vi "Error Query.vi"(6 "Ignored Warnings":string[](array[string]), 7 "Warnings as Errors":string[](array[string]), 8 "error in (no error)":errorcluster, 9 "Device and Axis":string, 10 "Previous Response Bundle Array":T1(array[cluster]), 11 "VISA resource name":refnum<visa-resource-name>) -> (0 "error out":errorcluster, 1 "Error Message":string, 2 "Error Code":i32, 3 "VISA resource name out":refnum<visa-resource-name>)   [LabVIEW 2015, in "Zaber A Series.lvlib"]
doc: "Checks a collection of responses for warning flags and reports all warnings from responding devices that have warning conditions.\n\nOptional inputs allow for ignoring some warnings or treating some warnings as error conditions. Both of these inputs are arrays of strings, each of which should be a two-letter warning code as seen in the Zaber ASCII Protocol Manual at http://www.zaber.com/wiki/Manuals/ASCII_Protocol_Manual#Warning_Flags. \n\nYou can globally ignore warnings or treat warnings as errors without having to wire up the relevant inputs everywhere by entering new defaults for the inputs - see the note on this VI's front panel.\n\nThis VI requires that the Initialize VI has been called with the same serial port."
uses:
  Zaber A Series.lvlib
  Private/All Commands.ctl
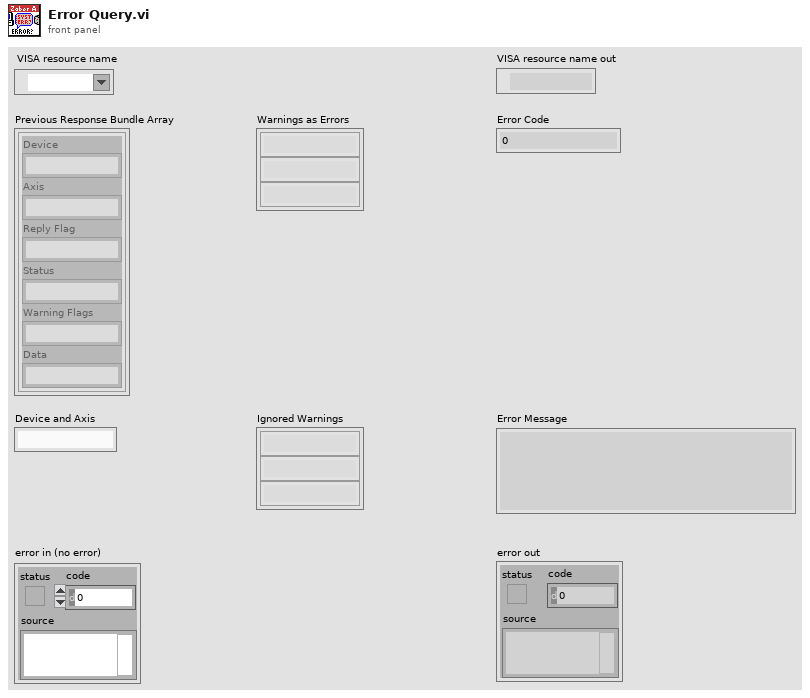
[diagram p1: front panel]
types:
  T1 = cluster{"Device":string, "Axis":string, "Reply Flag":string, "Status":string, "Warning Flags":string, "Data":string}[]
  T2 = typedef "Zaber A Series.lvlib/All Commands.ctl" = string
  T3 = cluster{"Device":string, "Axis":string, "Reply Flag":string, "Status":string, "Warning Flags":string, "Data":string}
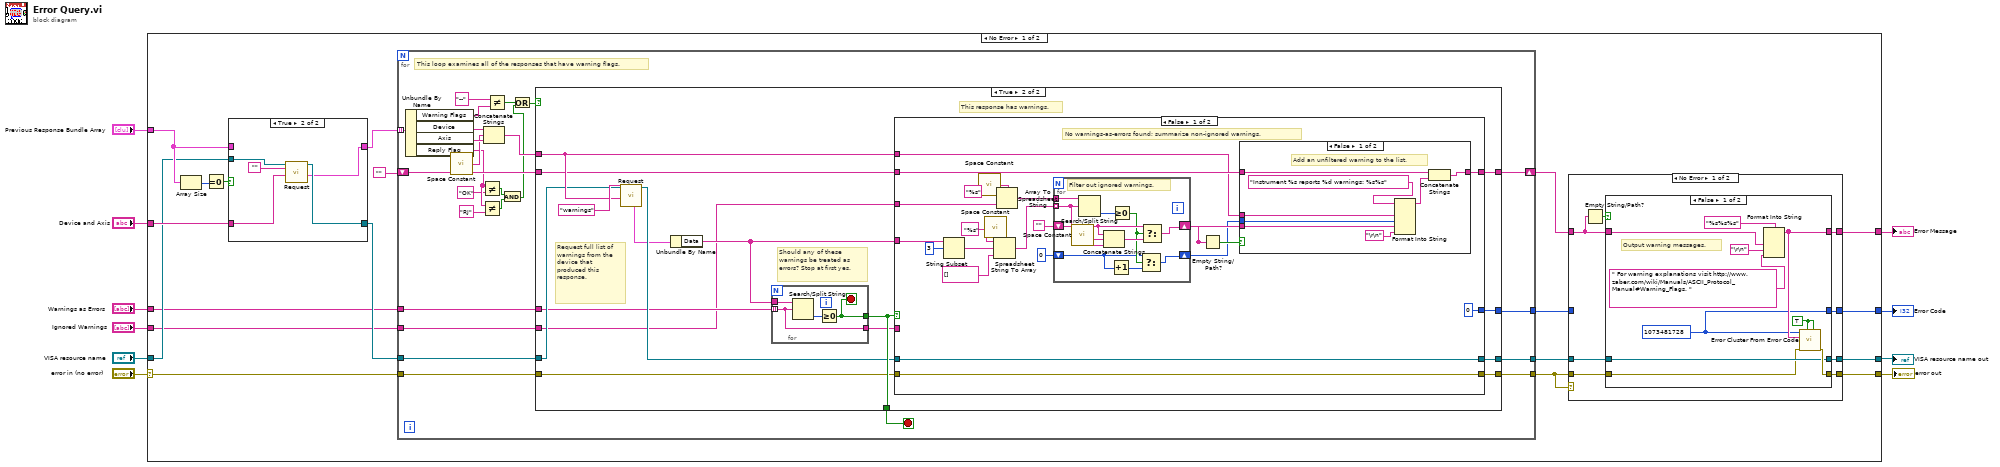
[diagram p0: block diagram]
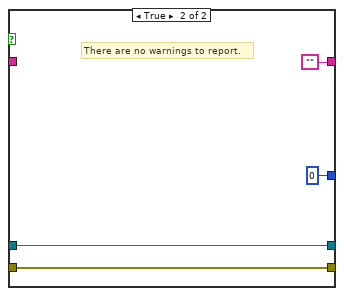
[diagram p3: hidden frame]
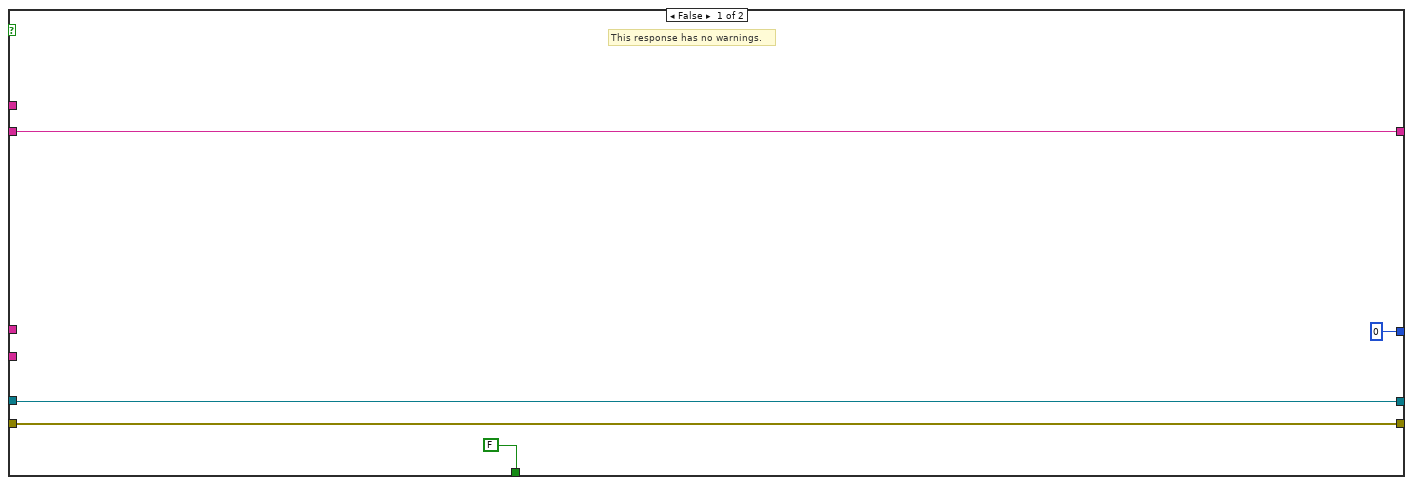
[diagram p5: hidden frame]
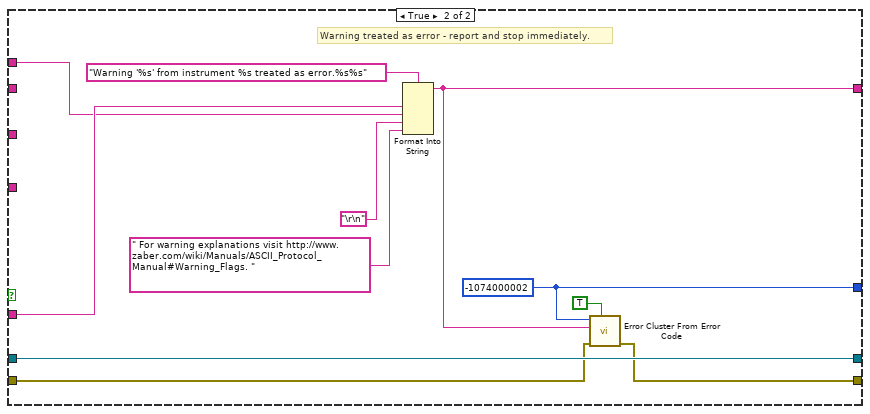
[diagram p7: hidden frame]
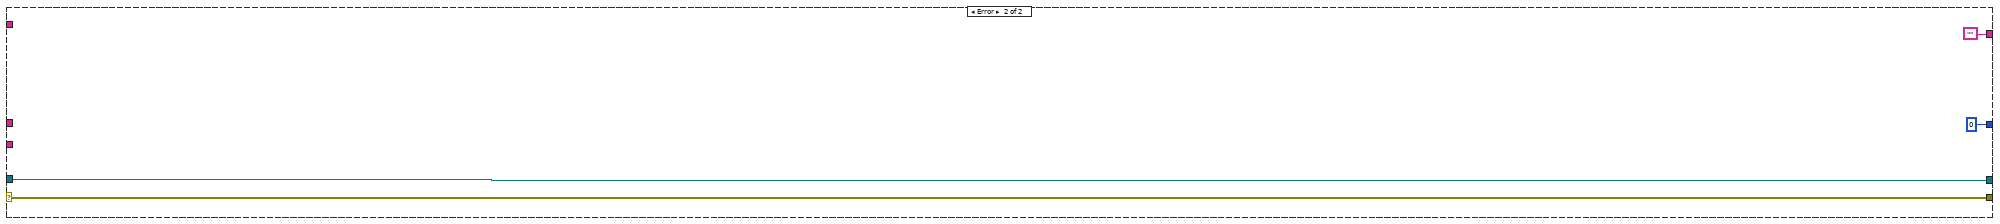
[diagram p8: hidden frame]
diagram:
  n1 = case shown="No Error" "error in (no error)" {
    selector: "error in (no error)" -> [w25 w168]
    tunnel: [w27 w169] -> w10
    tunnel: "VISA resource name" -> [w14 w169]
    tunnel: [w28 w168] -> w6
    tunnel: [w26 ""] -> w4
    tunnel: [w29 0 ("Code")] -> w7
    tunnel: "Device and Axis" -> [w15 _]
    tunnel: "Previous Response Bundle Array" -> [w17 _]
    tunnel: "Warnings as Errors" -> [w12 _]
    tunnel: "Ignored Warnings" -> [w11 _]
    frame No Error {
      n2 = Array Size(array=w17) -> (size(s)=w24:i32)
      n3 = Equal To 0?(x=w24) -> (x = 0?=w18:bool)
      n4 = case shown="True" w18 {
        tunnel: w17 -> [w31 _]
        tunnel: [w31 w32] -> w16
        tunnel: w15 -> [_ w36]
        tunnel: w14 -> [w30 w34]
        tunnel: [w30 w33] -> w13
        frame False {
        }
        frame True {
          n5 = call "Request.vi"("Device and Axis"=w36, "Command String"="", "VISA resource name"=w34) -> ("Response Bundle Array"=w32:T1, "VISA resource name out"=w33:refnum<visa-resource-name>)  [unwired: 3 in, 4 out]
        }
      }
      n6 = for {
        tunnel: w25 -> [w83]
        tunnel: [w87] -> w20
        tunnel: w16 -> [w82] mode=indexing
        tunnel: w13 -> [w85]
        tunnel: [w84] -> w21
        shift-right: [w73] -> w23
        shift-left: "" -> [w74]
        tunnel: [w86] -> w19
        tunnel: w12 -> [w64]
        tunnel: w11 -> [w63]
        stop <- w75 stop-if-true
        # "This loop examines all of the responses that have warning flags."
        n7 = Unbundle By Name(w82) -> ("Warning Flags"=w80:string, "Device"=w79:string, "Axis"=w78:string, "Reply Flag"=w72:string)
        n8 = call <vilib>:"Space Constant.vi"() -> ("String"=w77:string)
        n9 = Not Equal?(x=w72, y="OK") -> (x != y?=w69:bool)
        n10 = Not Equal?(x=w72, y="RJ") -> (x != y?=w68:bool)
        n11 = Concatenate Strings(w79, w77, w78) -> (w76:string)
        n12 = Not Equal?(x="--", y=w80) -> (x != y?=w66:bool)
        n13 = And(x=w69, y=w68) -> (x .and. y?=w65:bool)
        n14 = Or(x=w66, y=w65) -> (x .or. y?=w67:bool)
        n15 = case shown="True" w67 {
          tunnel: [w92 w108] -> w87
          tunnel: [0 ("error code (0)") w103] -> w86
          tunnel: w85 -> [w91 w96]
          tunnel: [w91 w104] -> w84
          tunnel: w83 -> [w92 w98]
          tunnel: w76 -> [_ w101]
          tunnel: [FALSE w106] -> w75
          tunnel: w74 -> [w89 w99]
          tunnel: [w89 w97] -> w73
          tunnel: w64 -> [_ w94]
          tunnel: w63 -> [_ w93]
          frame False {
            # "This response has no warnings."
          }
          frame True {
            # "This response has warnings."
            # "Should any of these warnings be treated as errors? Stop at first yes."
            # "Request full list of warnings from the device that produced this response."
            n16 = call "Request.vi"("Device and Axis"=w101, "Command String"=T2 "warnings" ("Warning Command"), "VISA resource name"=w96) -> ("VISA resource name out"=w105:refnum<visa-resource-name>, "First Response Bundle"=w95:T3)  [unwired: 3 in, 4 out]
            n17 = Unbundle By Name(w95) -> ("Data"=w100:string)
            n18 = for {
              tunnel: w94 -> [w109] mode=indexing
              tunnel: w100 -> [w112]
              tunnel: [w110] -> w106
              tunnel: [w109] -> w102
              stop <- w110 stop-if-true
              n19 = Search/Split String(string=w112, search string/char (-)=w109) -> (offset of match=w111:i32)  [unwired: 1 in, 2 out]
              n20 = Greater Or Equal To 0?(x=w111) -> (x >= 0?=w110:bool)
            }
            n21 = case shown="False" w106 {
              tunnel: [w132 w164] -> w108
              tunnel: [0 ("error code (0)") w163] -> w103
              tunnel: w98 -> [w132 w155]
              tunnel: w105 -> [w133 w165]
              tunnel: [w133 w165] -> w104
              tunnel: w102 -> [_ w160]
              tunnel: w101 -> [w118 w159]
              tunnel: w100 -> [w131 _]
              tunnel: w99 -> [w119 _]
              tunnel: [w115 w156] -> w97
              tunnel: w93 -> [w113 _]
              frame False {
                # "No warnings-as-errors found; summarize non-ignored warnings."
                n22 = String Subset(string=w131, offset (0)=3) -> (substring=w128:string)  [unwired: 1 in]
                n23 = call <vilib>:"Space Constant.vi"() -> ("String"=w130:string)
                n24 = call <vilib>:"Space Constant.vi"() -> ("String"=w126:string)
                n25 = Spreadsheet String To Array(delimiter (Tab)=w126, format string="%s", spreadsheet string=w128, array type (2D Dbl)=string[] []) -> (array=w124:string[])
                n26 = Array To Spreadsheet String(delimiter (Tab)=w130, array=w113, 3:"%s" ("format string")) -> (spreadsheet string=w123:string)
                n27 = for {
                  tunnel: w124 -> [w148] mode=indexing
                  tunnel: w123 -> [w154]
                  shift-right: [w151] -> w120
                  shift-left: "" -> [w150]
                  shift-right: [w146] -> w116
                  shift-left: 0 -> [w144]
                  # "Filter out ignored warnings."
                  n28 = call <vilib>:"Space Constant.vi"() -> ("String"=w149:string)
                  n29 = Search/Split String(string=w154, search string/char (-)=w148) -> (offset of match=w153:i32)  [unwired: 1 in, 2 out]
                  n30 = Concatenate Strings(w150, w149, w148) -> (w152:string)
                  n31 = Increment(x=w144) -> (x+1=w145:i32)
                  n32 = Greater Or Equal To 0?(x=w153) -> (x >= 0?=w147:bool)
                  n33 = Select(t=w144, s=w147, f=w145) -> (s? t:f=w146:i32)
                  n34 = Select(t=w150, s=w147, f=w152) -> (s? t:f=w151:string)
                }
                n35 = Empty String/Path?(string/path=w120) -> (empty?=w121:bool)
                n36 = case shown="False" w121 {
                  tunnel: w120 -> [w138 _]
                  tunnel: [w136 w143] -> w115
                  tunnel: w119 -> [w141 w143]
                  tunnel: w118 -> [w140 _]
                  tunnel: w116 -> [w137 _]
                  frame False {
                    # "Add an unfiltered warning to the list."
                    n37 = Format Into String(format string="Instrument %s reports %d warnings: %s%s", w140, w137, w138, "\r\n") -> (resulting string=w142:string)  [unwired: 2 in, 1 out]
                    n38 = Concatenate Strings(w141, w142) -> (w136:string)
                  }
                  frame True {
                    # "No unfiltered warnings from this device."
                  }
                }
              }
              frame True {
                w163 = -1074000002 ("error code (0)")
                # "Warning treated as error - report and stop immediately."
                n39 = Format Into String(format string="Warning '%s' from instrument %s treated as error.%s%s", w160, w159, "\r\n", " For warning explanations visit http://www.zaber.com/wiki/Manuals/ASCII_Protocol_Manual#Warning_Flags. " ("string")) -> (resulting string=w156:string)  [unwired: 2 in, 1 out]
                n40 = call <vilib>:"Error Cluster From Error Code.vi"("show call chain? (False)"=TRUE, "error in (no error)"=w155, "error message (\"\")"=w156, "error code (0)"=w163) -> ("error out"=w164:errorcluster)  [unwired: 5 in]
              }
            }
          }
        }
      }
      n41 = case shown="No Error" w20 {
        tunnel: w21 -> [w39 w62]
        tunnel: [w38 w62] -> w27
        tunnel: w20 -> [w40 w61]
        tunnel: [w43 w61] -> w28
        tunnel: w19 -> [_ w59]
        tunnel: w23 -> [w42 w60]
        tunnel: [w44 w60] -> w26
        tunnel: [w37 w59] -> w29
        frame No Error {
          n42 = Empty String/Path?(string/path=w42) -> (empty?=w41:bool)
          n43 = case shown="False" w41 {
            tunnel: [w50 ""] -> w44
            tunnel: [w49 w58] -> w43
            tunnel: w42 -> [w48 _]
            tunnel: w40 -> [w46 w58]
            tunnel: w39 -> [w47 w57]
            tunnel: [w47 w57] -> w38
            tunnel: [w45 0 ("Code")] -> w37
            frame False {
              w45 = 1073481728 ("Code")
              w54 = TRUE ("show call chain? (False)")
              # "Output warning messages."
              n44 = Format Into String(format string="%s%s%s", w48, "\r\n", " For warning explanations visit http://www.zaber.com/wiki/Manuals/ASCII_Protocol_Manual#Warning_Flags. " ("string")) -> (resulting string=w50:string)  [unwired: 2 in, 1 out]
              n45 = call <vilib>:"Error Cluster From Error Code.vi"("is warning? (False)"=w54, "show call chain? (False)"=w54, "error in (no error)"=w46, "error message (\"\")"=w50, "error code (0)"=w45) -> ("error out"=w49:errorcluster)  [unwired: 4 in]
            }
            frame True {
              # "There are no warnings to report."
            }
          }
        }
        frame Error {
          # "In this case the error message and code outputs\nare only set if this VI generated the error."
          # "An error has already been generated; do not report warnings."
        }
      }
    }
    frame Error {
    }
  }
  "VISA resource name out" <- w10
  "Error Message" <- w4
  "Error Code" <- w7
  "error out" <- w6
